vi "_MAIN - Subpanel Demo.vi"() -> ()   [LabVIEW 2014]
uses:
  Flex UI (Parent)/Enum - Datum.ctl
  <vilib>/Utility/miscctls.llb/LVPositionTypeDef.ctl
  Flex UI Subpanel/Enum - Sizing.ctl
  Flex UI Subpanel/Flex UI Subpanel.lvclass
  Flex UI Dialog/Enum - Launch Position.ctl
  Flex UI (Parent)/Flex UI.lvclass
  Flex UI Dialog/Flex UI Dialog.lvclass
panel:
  in  "Embed":bool
  in  "Pop Out":bool
  in  "Sizing":T1
  in  "Cleanup":bool
  in  "Launch":bool
  in  "Position Settings":T4
  in  "Minimize":bool
  in  "Maximize":bool
  in  "Hide":bool
  in  "Show":bool
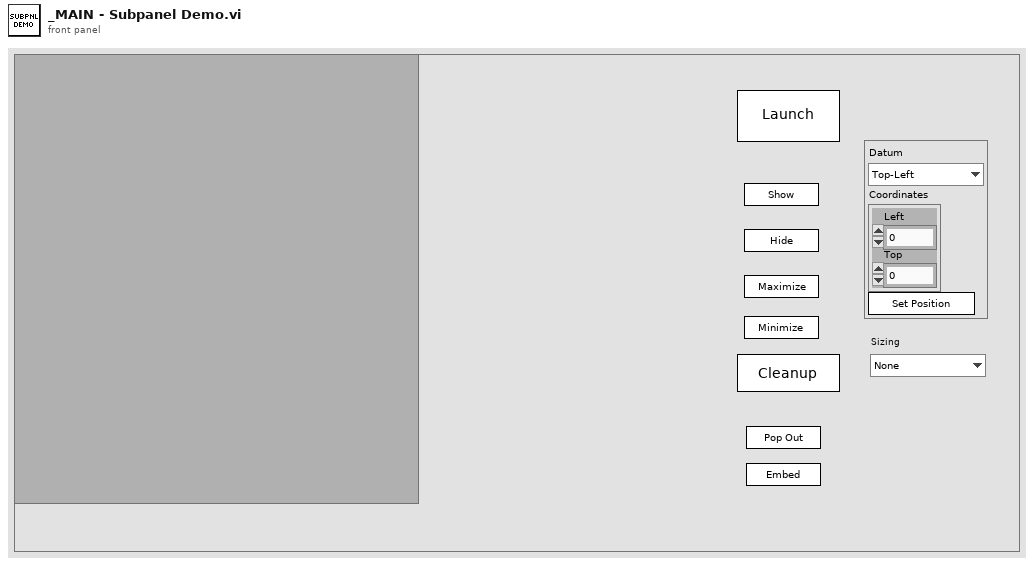
[diagram p1: front panel]
types:
  T1 = typedef "Flex UI Subpanel.lvclass/Enum - Sizing.ctl" = enum16{"None", "Largest Decoration", "Maximize"}
  T2 = typedef "Flex UI.lvclass/Enum - Datum.ctl" = enum16{"Top-Left", "Top-Right", "Bottom-Left", "Bottom-Right", "Center"}
  T3 = typedef "LVPositionTypeDef.ctl" = cluster{"Left":i32, "Top":i32}
  T4 = cluster{"Datum":T2, "Coordinates":T3, "Set Position":bool}
  T5 = typedef "Flex UI Dialog.lvclass/Enum - Launch Position.ctl" = enum16{"Default (Last Opened)", "Centered", "Centered on Caller", "Maximized", "Hidden"}
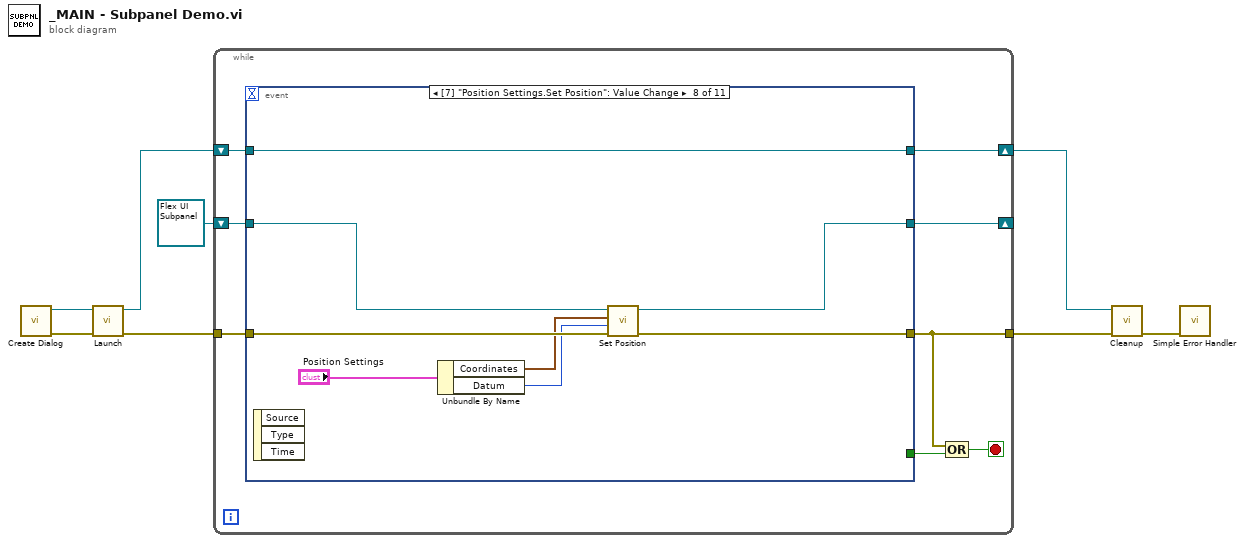
[diagram p0: block diagram]
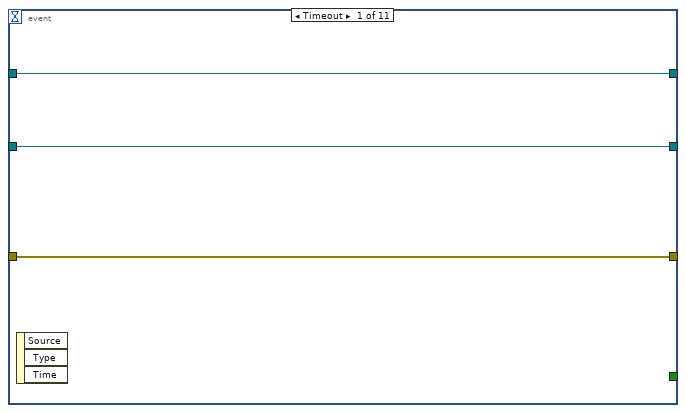
[diagram p2: hidden frame]
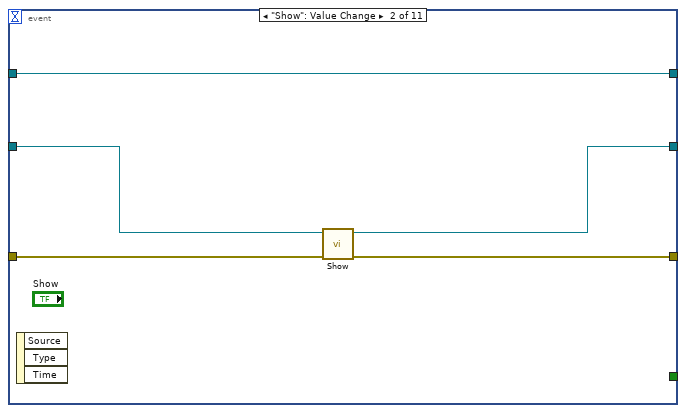
[diagram p3: hidden frame]
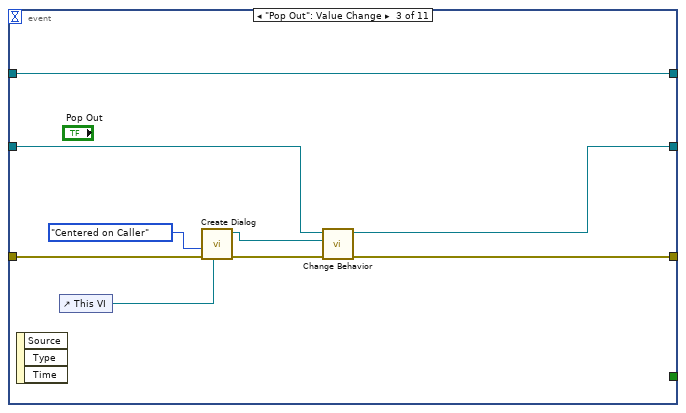
[diagram p4: hidden frame]
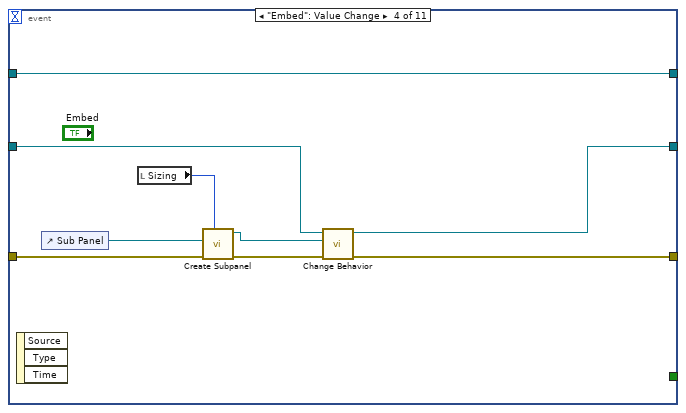
[diagram p5: hidden frame]
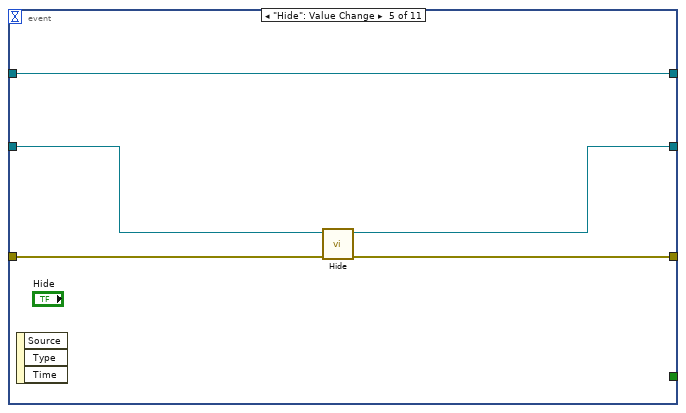
[diagram p6: hidden frame]
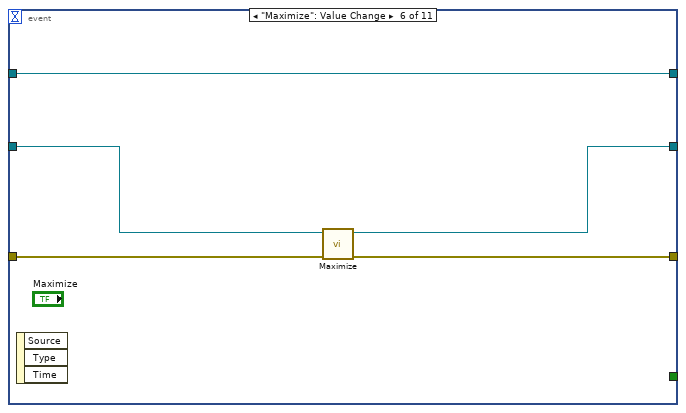
[diagram p7: hidden frame]
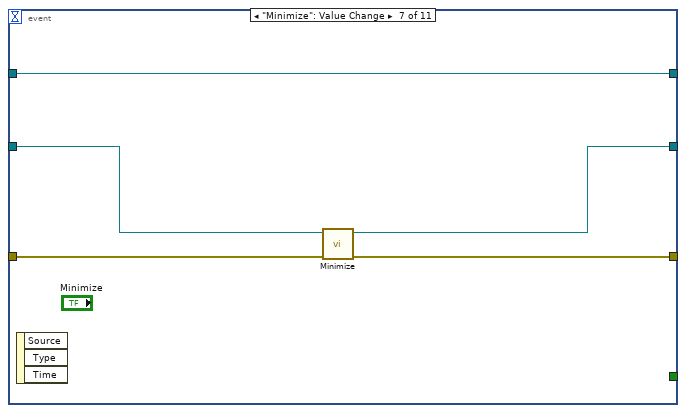
[diagram p8: hidden frame]
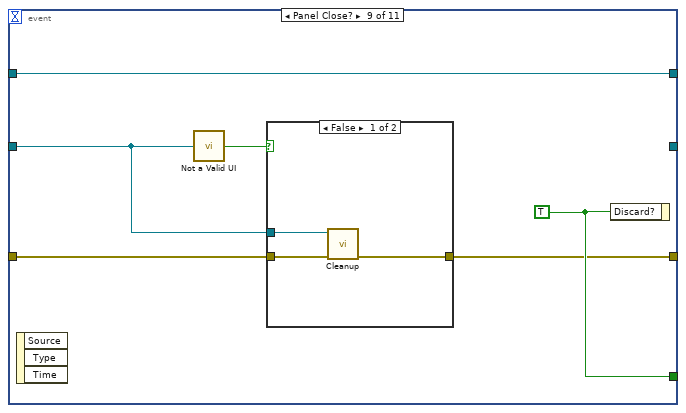
[diagram p9: hidden frame]
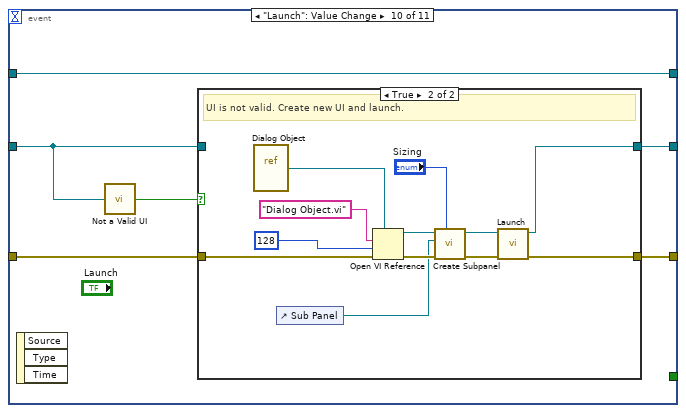
[diagram p11: hidden frame]
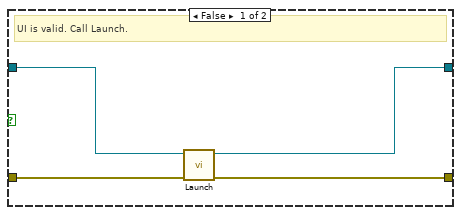
[diagram p12: hidden frame]
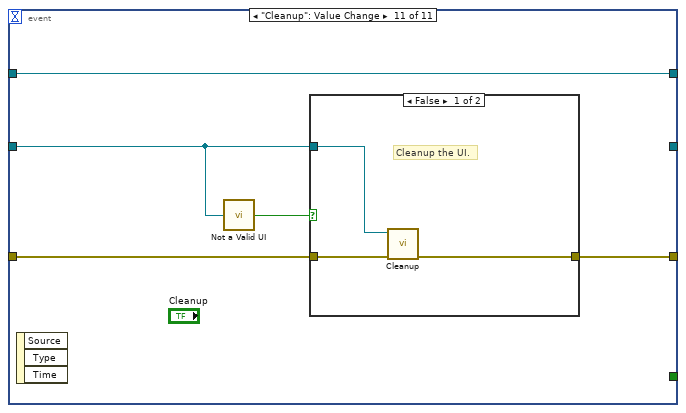
[diagram p13: hidden frame]
diagram:
  n1 = call "Create Dialog.vi"() -> ("error out"=w8:errorcluster, "Philips Dialog out"=w6:refnum<class "Flex UI Dialog.lvclass">)  [unwired: 10 in]
  n2 = call-dynamic "Launch.vi"("error in"=w8, "Philips Dialog in"=w6) -> ("error out"=w7:errorcluster, "Philips Dialog out"=w5:refnum<class "Flex UI Dialog.lvclass">)  [unwired: 8 in]
  n3 = while {
    tunnel: w7 -> [w14]
    shift-right: [w16] -> w4
    shift-left: w5 -> [w15]
    tunnel: [w11] -> w3
    shift-right: [w10] -> _
    shift-left: refnum<class "Flex UI Subpanel.lvclass"> refnum ("Philips Dialog out") -> [w9]
    stop <- w12 stop-if-true
    n4 = event shown="[7] \"Position Settings.Set Position\": Value Change" {
      selector: _ -> [_ _ _ _ _ _ _ _ _ _ _]
      dyn-events: _ -> [_ _ _ _ _ _ _ _ _ _ _]
      timeout: _ -> [_ _ _ _ _ _ _ _ _ _ _]
      tunnel: [w19 w24 w33 w41 w47 w52 w57 w65 w71 w81 w102] -> w16
      tunnel: w15 -> [w19 w24 w33 w41 w47 w52 w57 w65 w71 w81 w102]
      tunnel: w14 -> [w18 w20 w29 w42 w43 w48 w53 w61 w70 w80 w100]
      tunnel: [w18 w21 w30 w38 w44 w49 w54 w62 w68 w79 w101] -> w11
      tunnel: [_ _ _ _ _ _ _ _ w69 _ _] -> w13
      tunnel: [w17 w23 w32 w40 w46 w51 w56 w64 _ w78 _] -> w10
      tunnel: w9 -> [w17 w22 w31 w39 w45 w50 w55 w63 w67 w77 w99]
      event Timeout {
        n5 = event-data() -> ()  [unwired: 1 in, 3 out]
      }
      event "Show": Value Change {
        n6 = event-data() -> ()  [unwired: 1 in, 3 out]
        n7 = call-dynamic "Show.vi"("error in"=w20, "Philips UI in"=w22) -> ("error out"=w21:errorcluster, "Philips UI out"=w23:refnum<class "Flex UI.lvclass">)  [unwired: 8 in]
      }
      event "Pop Out": Value Change {
        n8 = event-data() -> ()  [unwired: 1 in, 3 out]
        n9 = control-ref of="This VI"() -> (w26:refnum<vi>)
        n10 = call "Create Dialog.vi"("Calling VI Reference"=w26, "error in"=w29, "Launch Position (Centered)"=Enum_-_Launch_Position."Centered on Caller") -> ("error out"=w28:errorcluster, "Philips Dialog out"=w27:refnum<class "Flex UI Dialog.lvclass">)  [unwired: 7 in]
        n11 = call "Change Behavior.vi"("error in"=w28, "New Behavior"=w27, "Philips UI in"=w31) -> ("error out"=w30:errorcluster, "New Behavior"=w32:refnum<class "Flex UI Dialog.lvclass">)  [unwired: 7 in]
      }
      event "Embed": Value Change {
        n12 = event-data() -> ()  [unwired: 1 in, 3 out]
        n13 = control-ref of="Sub Panel"() -> (w34:refnum<vi>)
        n14 = local read "Sizing"() -> (w35:T1)
        n15 = call "Create Subpanel.vi"("Sizing"=w35, "error in"=w42, "Subpanel Ref"=w34) -> ("error out"=w36:errorcluster, "Philips Subpanel out"=w37:refnum<class "Flex UI Subpanel.lvclass">)  [unwired: 7 in]
        n16 = call "Change Behavior.vi"("error in"=w36, "New Behavior"=w37, "Philips UI in"=w39) -> ("error out"=w38:errorcluster, "New Behavior"=w40:refnum<class "Flex UI Subpanel.lvclass">)  [unwired: 7 in]
      }
      event "Hide": Value Change {
        n17 = event-data() -> ()  [unwired: 1 in, 3 out]
        n18 = call-dynamic "Hide.vi"("error in"=w43, "Philips UI in"=w45) -> ("error out"=w44:errorcluster, "Philips UI out"=w46:refnum<class "Flex UI.lvclass">)  [unwired: 8 in]
      }
      event "Maximize": Value Change {
        n19 = event-data() -> ()  [unwired: 1 in, 3 out]
        n20 = call-dynamic "Maximize.vi"("error in"=w48, "Philips UI in"=w50) -> ("error out"=w49:errorcluster, "Philips UI out"=w51:refnum<class "Flex UI.lvclass">)  [unwired: 8 in]
      }
      event "Minimize": Value Change {
        n21 = event-data() -> ()  [unwired: 1 in, 3 out]
        n22 = call-dynamic "Minimize.vi"("error in"=w53, "Philips UI in"=w55) -> ("error out"=w54:errorcluster, "Philips UI out"=w56:refnum<class "Flex UI.lvclass">)  [unwired: 8 in]
      }
      event "Position Settings.Set Position": Value Change {
        n23 = event-data() -> ()  [unwired: 1 in, 3 out]
        n24 = Unbundle By Name("Position Settings") -> ("Coordinates"=w58:T3, "Datum"=w59:T2)
        n25 = call-dynamic "Set Position.vi"("error in"=w61, "Datum"=w59, "Target Coordinates"=w58, "Philips UI in"=w63) -> ("error out"=w62:errorcluster, "Philips UI out"=w64:refnum<class "Flex UI.lvclass">)  [unwired: 6 in]
      }
      event Panel Close? {
        w69 = TRUE ("Discard?")
        n26 = event-data() -> ()  [unwired: 1 in, 3 out]
        n27 = call "Not a Valid UI.vi"("Philips UI in"=w67) -> ("Not a Valid UI"=w66:bool)
        n28 = case shown="False" w66 {
          tunnel: w70 -> [w74 w75]
          tunnel: [w73 w75] -> w68
          tunnel: w67 -> [w72 _]
          frame False {
            n29 = call-dynamic "Cleanup.vi"("error in"=w74, "Philips UI in"=w72) -> ("error out"=w73:errorcluster)  [unwired: 9 in]
          }
          frame True {
          }
        }
        n30 = event-data("Discard?"=w69) -> ()  [unwired: 1 in, 1 out]
      }
      event "Launch": Value Change {
        n31 = event-data() -> ()  [unwired: 1 in, 3 out]
        n32 = call "Not a Valid UI.vi"("Philips UI in"=w77) -> ("Not a Valid UI"=w76:bool)
        n33 = case shown="True" w76 {
          tunnel: w80 -> [w85 w95]
          tunnel: [w84 w91] -> w79
          tunnel: [w82 w89] -> w78
          tunnel: w77 -> [w83 _]
          frame False {
            # "UI is valid. Call Launch."
            n34 = call-dynamic "Launch.vi"("error in"=w85, "Philips UI in"=w83) -> ("error out"=w84:errorcluster, "Philips UI out"=w82:refnum<class "Flex UI.lvclass">)  [unwired: 8 in]
          }
          frame True {
            # "UI is not valid. Create new UI and launch."
            n35 = vi-ref "Dialog Object.vi"() -> (w88:refnum<vi>)
            n36 = control-ref of="Sub Panel"() -> (w86:refnum<vi>)
            n37 = Open VI Reference(type specifier VI Refnum (for type only)=w88, vi path="Dialog Object.vi", options=128, error in (no error)=w95) -> (vi reference=w92:refnum<vi>, error out=w94:errorcluster)  [unwired: 2 in]
            n38 = call "Create Subpanel.vi"("Sizing"="Sizing", "error in"=w94, "Subpanel Ref"=w86, "UI VI Reference (caller)"=w92) -> ("error out"=w93:errorcluster, "Philips Subpanel out"=w90:refnum<class "Flex UI Subpanel.lvclass">)  [unwired: 6 in]
            n39 = call-dynamic "Launch.vi"("error in"=w93, "Philips Subpanel in"=w90) -> ("error out"=w91:errorcluster, "Philips Subpanel out"=w89:refnum<class "Flex UI Subpanel.lvclass">)  [unwired: 8 in]
          }
        }
      }
      event "Cleanup": Value Change {
        n40 = event-data() -> ()  [unwired: 1 in, 3 out]
        n41 = call "Not a Valid UI.vi"("Philips UI in"=w99) -> ("Not a Valid UI"=w98:bool)
        n42 = case shown="False" w98 {
          tunnel: [w105 w106] -> w101
          tunnel: w100 -> [w104 w106]
          tunnel: w99 -> [w103 _]
          frame False {
            # "Cleanup the UI."
            n43 = call-dynamic "Cleanup.vi"("error in"=w104, "Philips UI in"=w103) -> ("error out"=w105:errorcluster)  [unwired: 9 in]
          }
          frame True {
          }
        }
      }
    }
    n44 = Compound Arithmetic op=OR(w11, w13) -> (w12:bool)
  }
  n45 = call-dynamic "Cleanup.vi"("error in"=w3, "Philips Dialog in"=w4) -> ("error out"=w2:errorcluster)  [unwired: 9 in]
  n46 = call <vilib>:"Simple Error Handler.vi"("error in (no error)"=w2) -> ()  [unwired: 4 in, 5 out]
